vi "Modder.vi"() -> ()   [LabVIEW 2015]
doc: "Build a sequence for running an experiment. \n\nCreate a template VAR array on the sequence tab. This should be used to set any VAR values which will be static throughout an experiment. For VARS that will change during the experiment use a placeholder 'TAG', which can be any string that's unique in the XML file."
uses:
  oskar_tools/mod_tag.ctl
  oskar_tools/seq_line.ctl
  <vilib>/gmath/NI_Gmath.lvlib
  oskar_tools/oskar_tools.lvlib
panel:
  in  "Line":T1
  out "error out":errorcluster
  out "String Formats":string[](array[string])
  in  "Send Button":bool
  in  "Save Button":bool
  in  "Save":path
  in  "Stop Button":bool
  in  "Make Button":bool
  in  "Tab Control":enum32{"Sequence", "TAGS"}(tab)
  in  "Open Button":bool
  in  "Template SEQ":T1
  out "Output SEQs":T1[](array[typedef])
  out "Built":i32
  out "Progress":u8(slide)=100 max=15 scale=0.0..100.0 scale format="%.2f"
  in  "defualt format":string="%0.4g"
  in  "Reorder":bool
  out "TAGS":string[](array[string])
  out "TAG Permutations":dbl[][](array[numeric]) format="%#_8g"
  in  "Build Arrays":T2[](array[typedef]) {"Steps" min=1 step=1}
  out "size(s)":i32[](array[numeric])
  # "Modder"
  # "Use $math ($) to start (end) expressions,\ne.g. $math (XX +1 ) / XY $"
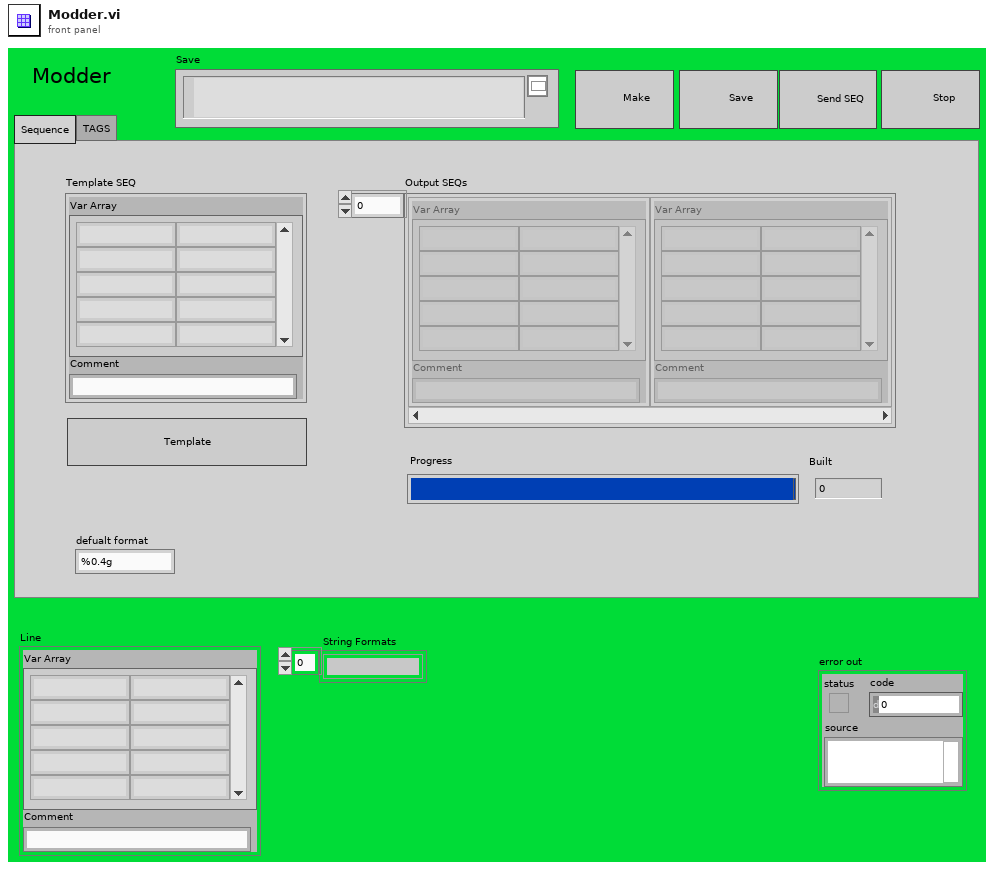
[diagram p1: front panel]
types:
  T1 = typedef "oskar_tools.lvlib/seq_line.ctl" = cluster{"Var Array":string[][], "Comment":string}
  T2 = typedef "oskar_tools.lvlib/mod_tag.ctl" = cluster{"TAG":string, "Array":dbl[], "f(x)":string, "Steps":i32, "Build":bool, "Reorder Each":bool, "Format":string}
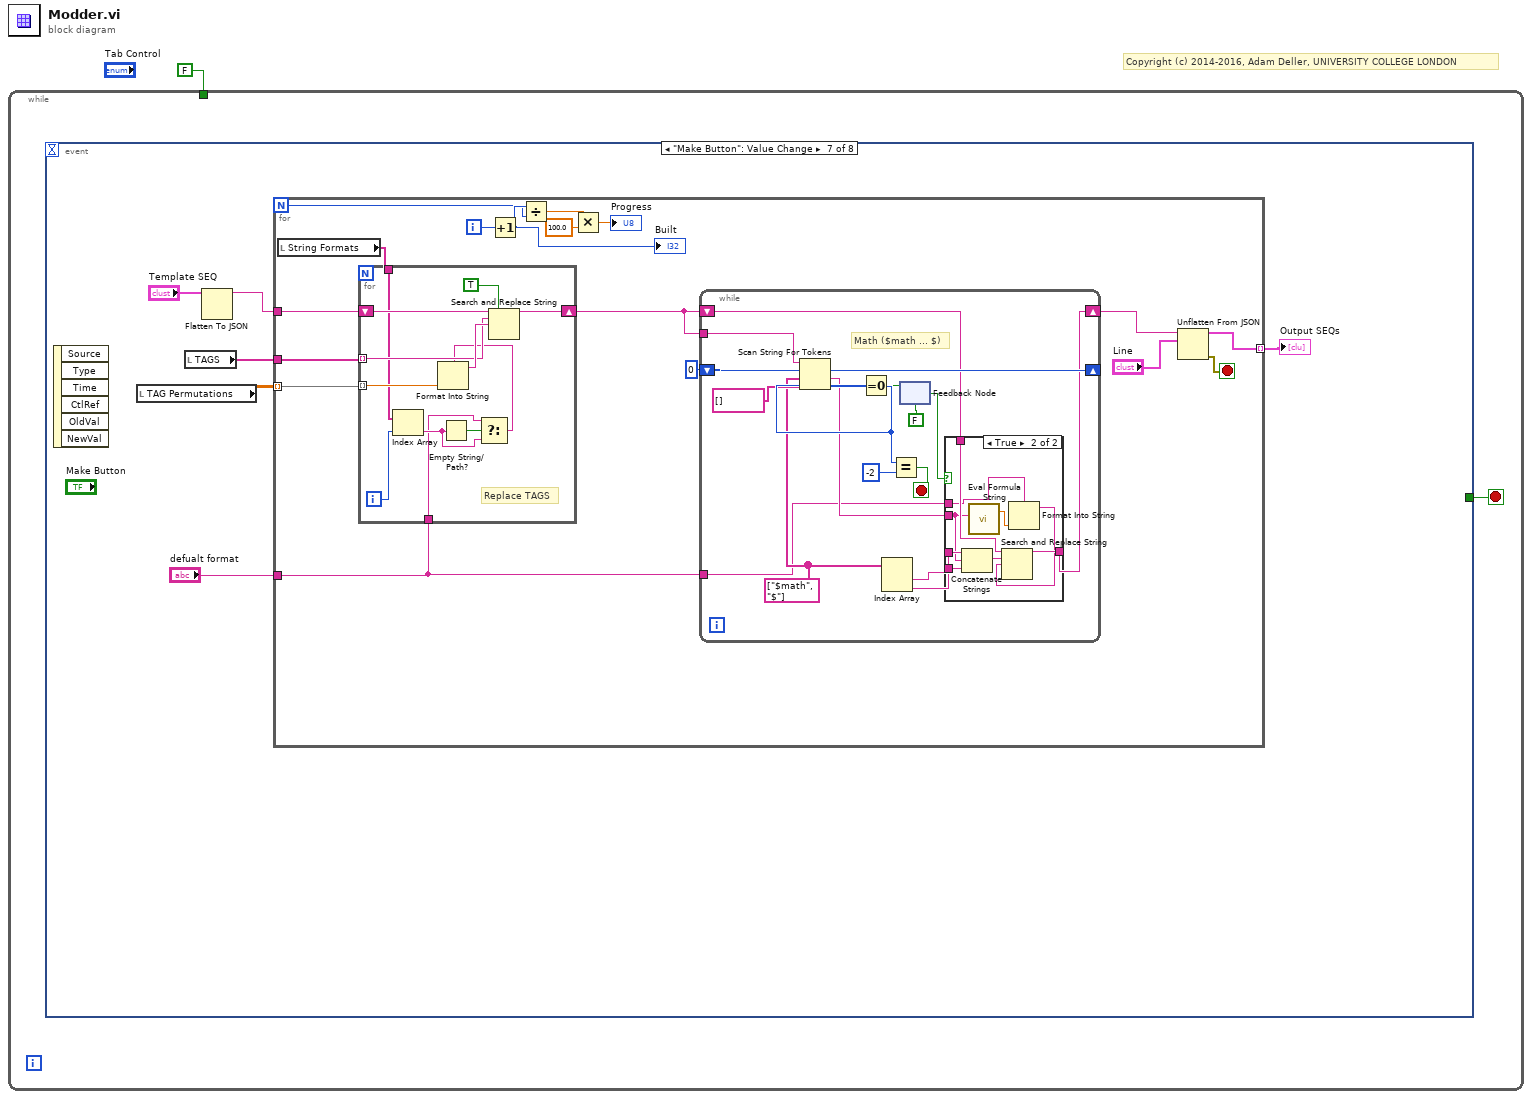
[diagram p0: block diagram]
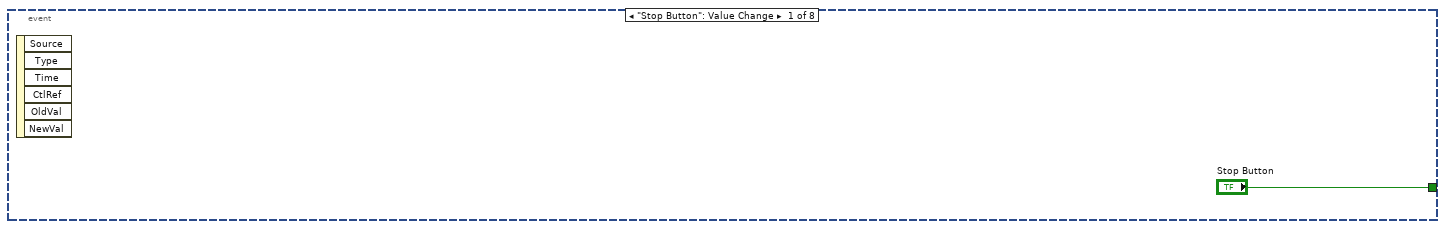
[diagram p2: hidden frame]
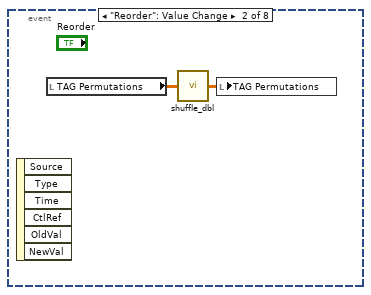
[diagram p3: hidden frame]
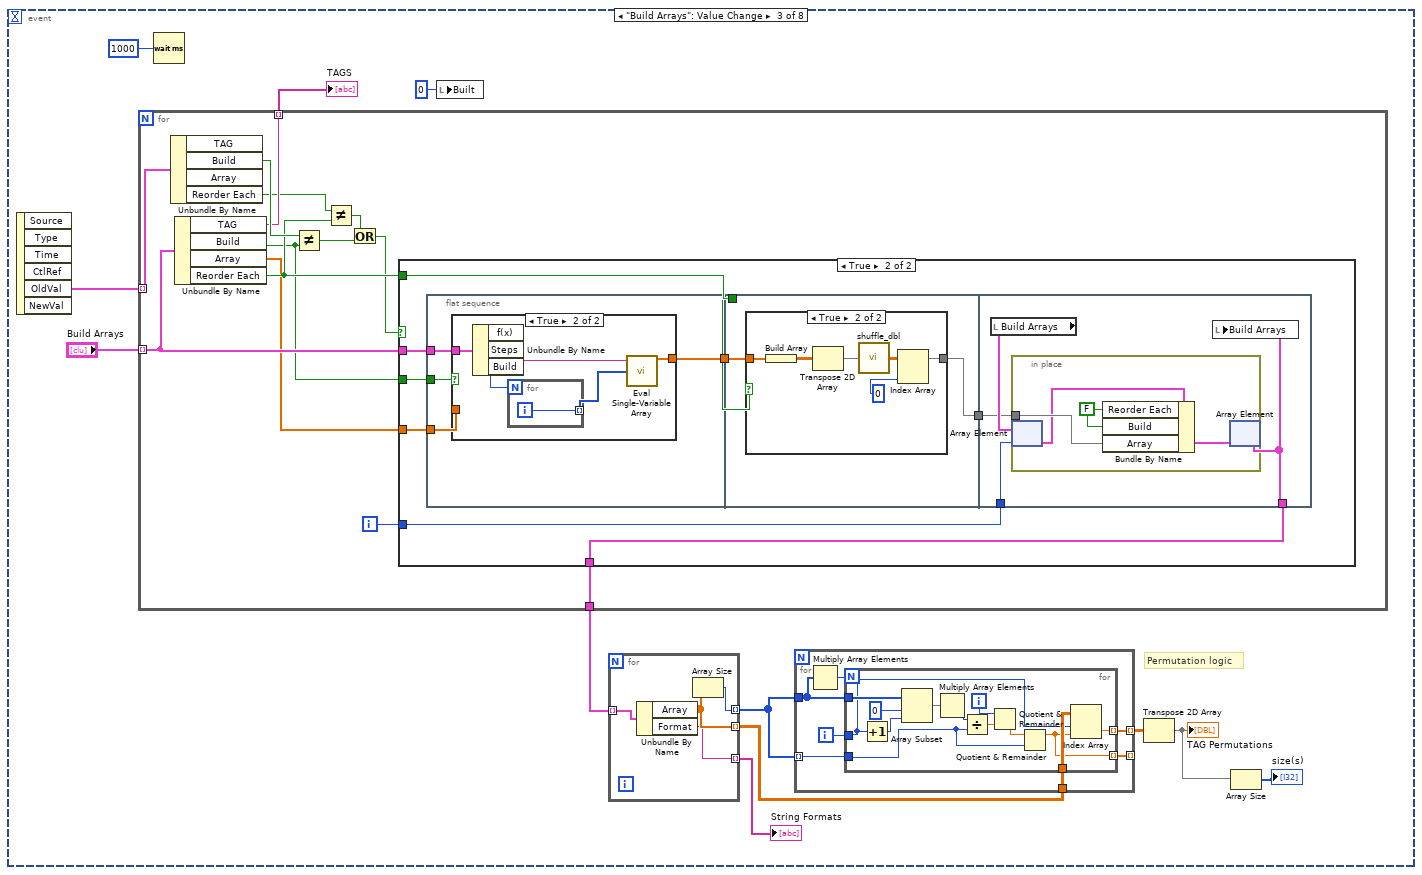
[diagram p4: hidden frame]
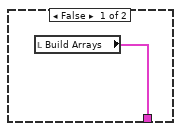
[diagram p5: hidden frame]
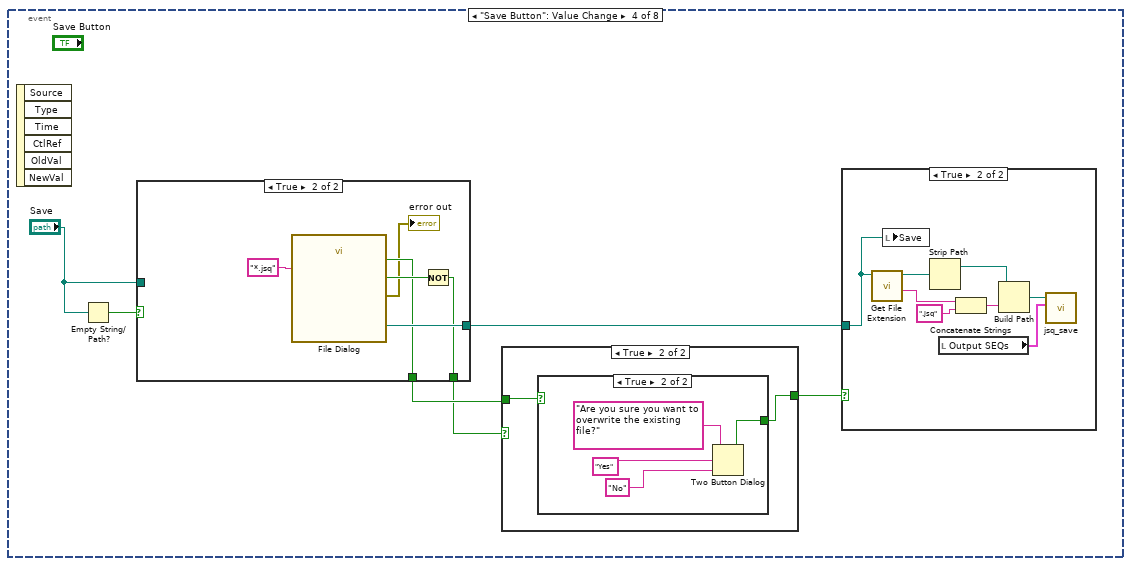
[diagram p8: hidden frame]
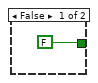
[diagram p9: hidden frame]
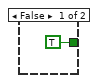
[diagram p10: hidden frame]
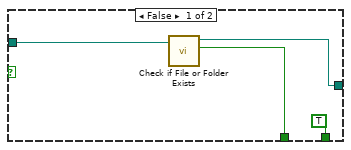
[diagram p11: hidden frame]
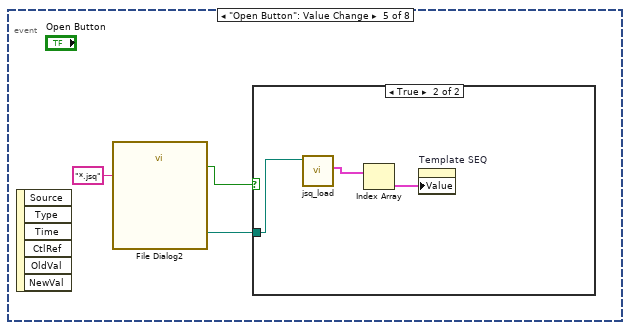
[diagram p13: hidden frame]
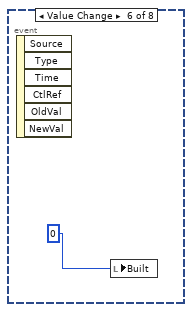
[diagram p15: hidden frame]
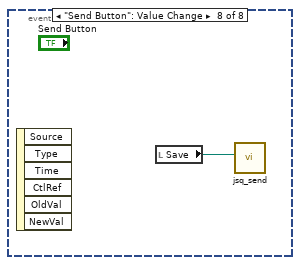
[diagram p17: hidden frame]
diagram:
  # "Copyright (c) 2014-2016, Adam Deller, UNIVERSITY COLLEGE LONDON"
  n1 = while {
    tunnel: FALSE ("Done") -> [_]
    stop <- w2 stop-if-true
    n2 = event shown="[6] \"Make Button\": Value Change" {
      selector: _ -> [_ _ _ _ _ _ _ _]
      dyn-events: _ -> [_ _ _ _ _ _ _ _]
      timeout: _ -> [_ _ _ _ _ _ _ _]
      tunnel: ["Stop Button" _ _ _ _ _ _ _] -> w2
      event "Stop Button": Value Change {
        n3 = event-data() -> ()  [unwired: 1 in, 6 out]
      }
      event "Reorder": Value Change {
        n4 = event-data() -> ()  [unwired: 1 in, 6 out]
        n5 = local read "TAG Permutations"() -> (w5:dbl[][])
        n6 = call "shuffle_dbl.vi"("Array IN"=w5) -> ("Array OUT"=w4:dbl[][])
        n7 = local write "TAG Permutations"(w4) -> ()
      }
      event "Build Arrays": Value Change {
        # "Permutation logic"
        n8 = event-data() -> ("OldVal"=w17:T2[])  [unwired: 1 in, 5 out]
        n9 = for {
          tunnel: "Build Arrays" -> [w53] mode=indexing
          tunnel: w17 -> [w54] mode=indexing
          tunnel: [w50] -> w15 mode=indexing
          tunnel: [w42] -> w9
          i -> [w52]
          n10 = Unbundle By Name(w54) -> ("Build"=w51:bool, "Reorder Each"=w49:bool)  [unwired: 2 out]
          n11 = Unbundle By Name(w53) -> ("TAG"=w50:string, "Build"=w43:bool, "Array"=w45:dbl[], "Reorder Each"=w48:bool)
          n12 = Not Equal?(x=w51, y=w43) -> (x != y?=w46:bool)
          n13 = Not Equal?(x=w49, y=w48) -> (x != y?=w47:bool)
          n14 = Or(x=w47, y=w46) -> (x .or. y?=w44:bool)
          n15 = case shown="True" w44 {
            tunnel: w53 -> [_ w63]
            tunnel: w52 -> [_ w62]
            tunnel: w45 -> [_ w57]
            tunnel: w48 -> [_ w60]
            tunnel: [w55 w58] -> w42
            tunnel: w43 -> [_ w56]
            frame False {
              n16 = local read "Build Arrays"() -> (w55:T2[])
            }
            frame True {
              n17 = flat-sequence {
                tunnel: w63 -> [w67]
                tunnel: [w66] -> w61
                tunnel: w57 -> [w65]
                tunnel: w56 -> [w64]
                tunnel: w61 -> [w76]
                tunnel: w60 -> [w77]
                tunnel: [w75] -> w59
                tunnel: w62 -> [w88]
                tunnel: [w85] -> w58
                tunnel: w59 -> [w86]
                frame #0 {
                  n18 = case shown="True" w64 {
                    tunnel: w67 -> [_ w73]
                    tunnel: [w68 w69] -> w66
                    tunnel: w65 -> [w68 _]
                    frame False {
                    }
                    frame True {
                      n19 = Unbundle By Name(w73) -> ("f(x)"=w72:string, "Steps"=w71:i32)  [unwired: 1 out]
                      n20 = for {
                        N: w71 -> [_]
                        tunnel: [w74] -> w70 mode=indexing
                        i -> [w74]
                      }
                      n21 = call <vilib>:"Eval Single-Variable Array.vi"("X Values"=w70, "formula"=w72) -> ("Y Values"=w69:dbl[])  [unwired: 1 in, 1 out]
                    }
                  }
                }
                frame #1 {
                  n22 = case shown="True" w77 {
                    tunnel: w76 -> [w78 w84]
                    tunnel: [w78 w82] -> w75
                    frame False {
                    }
                    frame True {
                      n23 = Build Array(w84) -> (w81:dbl[][])
                      n24 = Transpose 2D Array(2D array=w81) -> (transposed array=w80:dbl[][])
                      n25 = call "shuffle_dbl.vi"("Array IN"=w80) -> ("Array OUT"=w83:dbl[][])
                      n26 = Index Array(array=w83, index (col)=0 ("disabled index (col)")) -> (element=w82:dbl[])  [unwired: 1 in]
                    }
                  }
                }
                frame #2 {
                  n27 = local read "Build Arrays"() -> (w87:T2[])
                  n28 = in-place {
                    in-place-border: w86 -> [w92]
                    w89 = FALSE ("Use")
                    n29 = in-place-array #1(w87, w88) -> (w91:T2)
                    n30 = Bundle By Name(cluster=w91, "Reorder Each"=w89, "Build"=w89, "Array"=w92) -> (w90:T2)
                    n31 = in-place-array #1(w90) -> (w85:T2[])  [unwired: 1 out]
                  }
                  n32 = local write "Build Arrays"(w85) -> ()
                }
              }
            }
          }
        }
        "TAGS" <- w15
        n33 = Wait (ms)(milliseconds to wait=1000) -> ()  [unwired: 1 out]
        n34 = local write "Built"(0 ("Built")) -> ()
        n35 = for {
          tunnel: [w20] -> w10 mode=indexing
          tunnel: [w21] -> w11 mode=indexing
          tunnel: w9 -> [w19] mode=indexing
          tunnel: [w18] -> w6 mode=indexing
          n36 = Unbundle By Name(w19) -> ("Array"=w21:dbl[], "Format"=w18:string)
          n37 = Array Size(array=w21) -> (size(s)=w20:i32)
        }
        "String Formats" <- w6
        n38 = for {
          tunnel: w10 -> [w27]
          tunnel: w10 -> [w25] mode=indexing
          tunnel: w11 -> [w24]
          tunnel: [w23] -> w12 mode=indexing
          tunnel: [w22] -> _ mode=indexing
          i -> [w28]
          n39 = Multiply Array Elements(1:w27) -> (0:w26:i32)
          n40 = for {
            N: w26 -> [_]
            tunnel: w27 -> [w40]
            tunnel: w28 -> [w30]
            tunnel: w25 -> [w35]
            tunnel: w24 -> [w33]
            tunnel: [w32] -> w23 mode=indexing
            tunnel: [w29] -> w22 mode=indexing
            i -> [w31]
            n41 = Increment(x=w30) -> (x+1=w38:i32)
            n42 = Array Subset(array=w40, index=0, length=w38) -> (w39:i32[])
            n43 = Multiply Array Elements(1:w39) -> (0:w37:i32)
            n44 = Divide(x=w37, y=w35) -> (x/y=w36:dbl)
            n45 = Quotient & Remainder(x=w31, y=w36) -> (floor(x/y)=w34:dbl)  [unwired: 1 out]
            n46 = Quotient & Remainder(x=w34, y=w35) -> (x-y*floor(x/y)=w29:dbl)  [unwired: 1 out]
            n47 = Index Array(array=w33, index (row)=w30, index (col)=w29) -> (element=w32:dbl)
          }
        }
        n48 = Transpose 2D Array(2D array=w12) -> (transposed array=w8:dbl[][])
        "TAG Permutations" <- w8
        n49 = Array Size(array=w8) -> (size(s)=→"size(s)":i32[])
      }
      event "Save Button": Value Change {
        n50 = event-data() -> ()  [unwired: 1 in, 6 out]
        n51 = Empty String/Path?(string/path="Save") -> (empty?=w98:bool)
        n52 = case shown="True" w98 {
          tunnel: "Save" -> [w110 _]
          tunnel: [w108 w115] -> w93
          tunnel: [w109 w112] -> w97
          tunnel: [TRUE w113] -> w96
          frame False {
            n53 = call <vilib>:"Check if File or Folder Exists.vi"("path"=w110) -> ("file or folder exists?"=w109:bool, "dup path"=w108:path)  [unwired: 8 in, 1 out]
          }
          frame True {
            n54 = call "File Dialog"("pattern (all files)"="*.jsq") -> ("selected path"=w115:path, "exists"=w112:bool, "cancelled"=w114:bool, "error out"=→"error out":errorcluster)  [unwired: 11 in]
            n55 = Not(x=w114) -> (.not. x?=w113:bool)
          }
        }
        n56 = case shown="True" w96 {
          tunnel: w97 -> [_ w101]
          tunnel: [FALSE w100] -> w95
          frame False {
          }
          frame True {
            n57 = case shown="True" w101 {
              tunnel: [TRUE ("T button?") w104] -> w100
              frame False {
              }
              frame True {
                n58 = Two Button Dialog(message="Are you sure you want to overwrite the existing file?", 1:"No" ("Right Button Text (\"Cancel\")"), 2:"Yes" ("T button name (\"OK\")")) -> (T button?=w104:bool)
              }
            }
          }
        }
        n59 = case shown="True" w95 {
          tunnel: w93 -> [_ w117]
          frame False {
          }
          frame True {
            n60 = call <vilib>:"Get File Extension.vi"("file"=w117) -> ("filename without extension"=w121:string, "dup file"=w119:path)  [unwired: 6 in, 3 out]
            n61 = local write "Save"(w117) -> ()
            n62 = Strip Path(path=w119) -> (stripped path=w118:path)  [unwired: 1 out]
            n63 = local read "Output SEQs"() -> (w124:T1[])
            n64 = Concatenate Strings(w121, ".jsq" ("string")) -> (w122:string)
            n65 = Build Path(base path=w118, name or relative path=w122) -> (appended path=w120:path)
            n66 = call "jsq_save.vi"("SEQs"=w124, "Save"=w120) -> ()  [unwired: 8 in, 2 out]
          }
        }
      }
      event "Open Button": Value Change {
        n67 = event-data() -> ()  [unwired: 1 in, 6 out]
        n68 = call "File Dialog2"("pattern (all files)"="*.jsq") -> ("selected path"=w126:path, "exists"=w127:bool)  [unwired: 11 in, 2 out]
        n69 = case shown="True" w127 {
          tunnel: w126 -> [_ w130]
          frame False {
          }
          frame True {
            n70 = call "jsq_load.vi"("Open"=w130) -> ("SEQs"=w129:T1[])  [unwired: 7 in, 3 out]
            n71 = Index Array(array=w129) -> (element=w128:T1)  [unwired: 1 in]
            n72 = property on="Template SEQ" class="Clust (strict)"("Value"=w128) -> ()  [unwired: 2 in, 2 out]
          }
        }
      }
      event Value Change {
        n73 = event-data() -> ()  [unwired: 1 in, 6 out]
        n74 = local write "Built"(u8 0 ("Slide")) -> ()
      }
      event "Make Button": Value Change {
        n75 = event-data() -> ()  [unwired: 1 in, 6 out]
        n76 = local read "TAG Permutations"() -> (w137:dbl[][])
        n77 = local read "TAGS"() -> (w136:string[])
        n78 = Flatten To JSON(anything="Template SEQ") -> (JSON string=w134:string)  [unwired: 2 in, 1 out]
        n79 = for {
          N -> [w149]
          tunnel: w134 -> [w152]
          tunnel: w136 -> [w154]
          tunnel: w137 -> [w153] mode=indexing
          tunnel: [w145] -> w133 mode=indexing
          tunnel: "defualt format" -> [w140]
          i -> [w151]
          stop <- w144 stop-if-true
          n80 = local read "String Formats"() -> (w141:string[])
          n81 = for {
            tunnel: w154 -> [w188] mode=indexing
            tunnel: w153 -> [w193] mode=indexing
            shift-right: [w191] -> w142
            shift-left: w152 -> [w190]
            tunnel: w141 -> [w187]
            tunnel: w140 -> [w182]
            i -> [w186]
            # "Replace TAGS"
            n82 = Index Array(array=w187, index=w186) -> (element=w184:string)
            n83 = Empty String/Path?(string/path=w184) -> (empty?=w185:bool)
            n84 = Select(t=w182, s=w185, f=w184) -> (s? t:f=w183:string)
            n85 = Format Into String(format string=w183, w193) -> (resulting string=w189:string)  [unwired: 2 in, 1 out]
            n86 = Search and Replace String(replace all?=TRUE ("replace all? (F)"), input string=w190, search string=w188, replace string=w189) -> (result string=w191:string)  [unwired: 4 in, 3 out]
          }
          n87 = Increment(x=w151) -> (x+1=w150:i32)
          "Built" <- w150
          n88 = Divide(x=w150, y=w149) -> (x/y=w148:dbl)
          n89 = Multiply(x=w148, y=100.0) -> (x*y=→"Progress":dbl)
          n90 = while {
            shift-right: [w170] -> _
            shift-left: 0 ("offset past token") -> [w169]
            tunnel: w142 -> [w171]
            shift-right: [w156] -> w139
            shift-left: w142 -> [w157]
            tunnel: w140 -> [w155]
            stop <- w167 stop-if-true
            w161 = string[] ["$math", "$"] ("delimiters (\\s,\\t,\\r,\\n) 2")
            # "Math ($math ... $)"
            n91 = Scan String For Tokens(6:string[] [] ("delimiters (\\s,\\t,\\r,\\n)"), 7:w161, 8:w169, 9:w171) -> (0:w166:i32, 1:w158:string, 2:w170:i32)  [unwired: 2 in, 1 out]
            n92 = Equal To 0?(x=w166) -> (x = 0?=w165:bool)
            n93 = Index Array(array=w161) -> (element #1=w160:string, element #2=w159:string)  [unwired: 2 in]
            n94 = Equal?(x=w166, y=-2) -> (x = y?=w167:bool)
            n95 = feedback-in #2(w165) -> ()
            n96 = feedback #2(FALSE) -> (w162:bool)
            n97 = case shown="True" w162 {
              tunnel: w158 -> [_ w176]
              tunnel: w160 -> [_ w181]
              tunnel: w159 -> [_ w180]
              tunnel: w157 -> [w172 w178]
              tunnel: [w172 w177] -> w156
              tunnel: w155 -> [_ w173]
              frame False {
              }
              frame True {
                n98 = Concatenate Strings(w181, w176, w180) -> (w179:string)
                n99 = call <vilib>:"Eval Formula String.vi"("formula"=w176) -> ("y value"=w174:dbl)  [unwired: 1 in, 1 out]
                n100 = Format Into String(format string=w173, w174) -> (resulting string=w175:string)  [unwired: 2 in, 1 out]
                n101 = Search and Replace String(input string=w178, search string=w179, replace string=w175) -> (result string=w177:string)  [unwired: 5 in, 3 out]
              }
            }
          }
          n102 = Unflatten From JSON(JSON string=w139, type and defaults="Line") -> (value=w145:T1, error out=w144:errorcluster)  [unwired: 5 in]
        }
        "Output SEQs" <- w133
      }
      event "Send Button": Value Change {
        n103 = event-data() -> ()  [unwired: 1 in, 6 out]
        n104 = local read "Save"() -> (w194:path)
        n105 = call "jsq_send.vi"("Sequence File"=w194) -> ()  [unwired: 11 in]
      }
    }
  }
